vi "Compute ROI Grid v2.vi"(8 "Error In":errorcluster, 10 "Current ROI Bounds":T1, 11 "Grid Definition":T2) -> (0 "Error Out":errorcluster, 1 "ROI Names":string[](array[string]), 3 "Current ROI Descriptor":T4[](array[typedef]) {"Contours"."Type" items=["No Selection", "Point", "Line", "Rectangle", "Oval", "Polygon", "Freehand Region", "Annulus", "Unused2", "Unused3", "Broken Line", "Freehand Line", "Rotated Rectangle"]})   [LabVIEW 2021, in "Image.lvlib"]
uses:
  Image.lvlib
  ROI Grid Definition.ctl
  ROI  Type.ctl
  ROI Bounds.ctl
  <vilib>/Utility/error.llb/Error Cluster From Error Code.vi
  AlliGator/Globals, Variables, Constants/AlliGator Abort.vi
  <vilib>/ErrorRing/Error Ring.xnode
  AlliGator/Globals, Variables, Constants/AlliGator Globals, Variables & Constants.lvlib
  Utilities/Utilities.lvlib
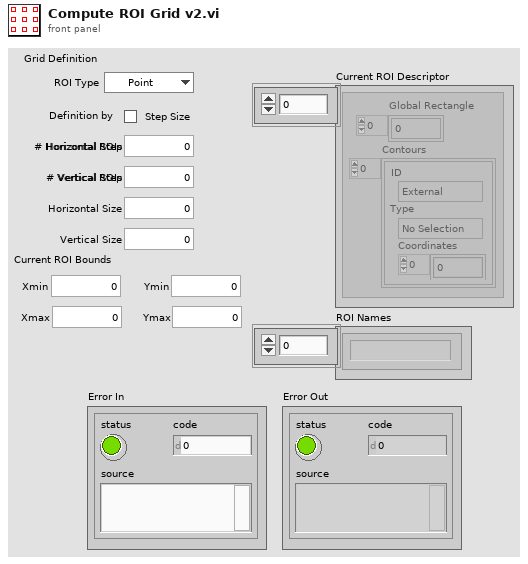
[diagram p1: front panel]
types:
  T1 = typedef "Image.lvlib/ROI Bounds.ctl" = cluster{"Ymax":i32, "Xmin":i32, "Ymin":i32, "Xmax":i32}
  T2 = typedef "Image.lvlib/ROI Grid Definition.ctl" = cluster{"Horizontal Step":i32, "Vertical Step":i32, "Horizontal Size":i32, "Vertical Size":i32, "# Horizontal ROIs":i32, "# Vertical ROIs":i32, "Definition by":bool, "ROI Type":T3}
  T3 = typedef "Image.lvlib/ROI  Type.ctl" = enum16{"Point", "Oval", "Rectangle"}
  T4 = typedef "ROI Descriptor" = cluster{"Global Rectangle":i32[], "Contours":cluster{"ID":enum32{"External", "Internal"}, "Type":u32, "Coordinates":i32[]}[]}
  T5 = typedef "IMAQ Rectangle" = cluster{"Left":i32, "Top":i32, "Right":i32, "Bottom":i32, "Rotation":dbl}
  T6 = typedef "IMAQ Point" = cluster{"X":sgl, "Y":sgl}
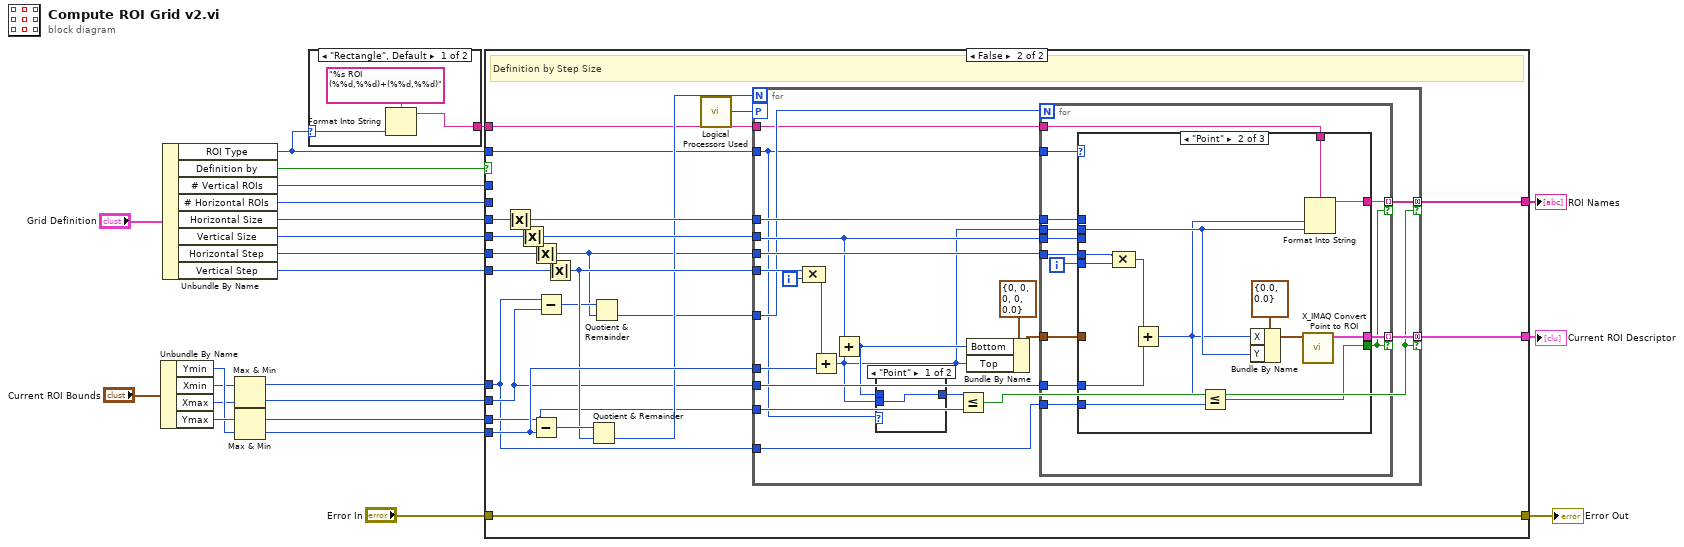
[diagram p0: block diagram]
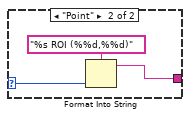
[diagram p2: hidden frame]
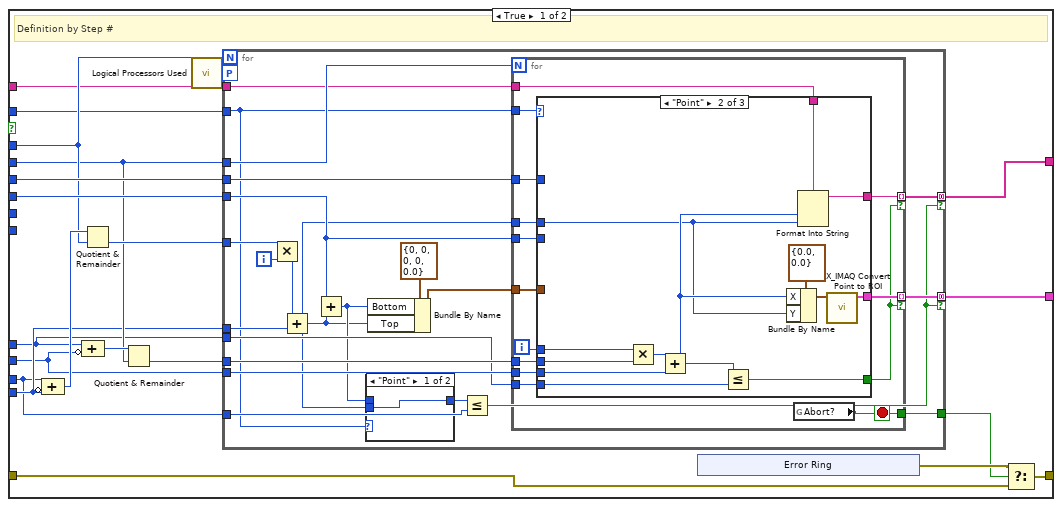
[diagram p3: hidden frame]
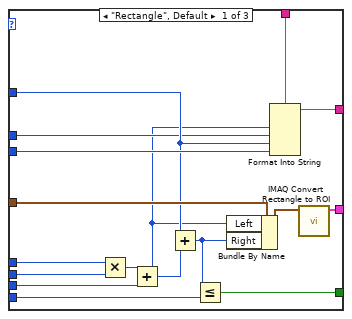
[diagram p5: hidden frame]
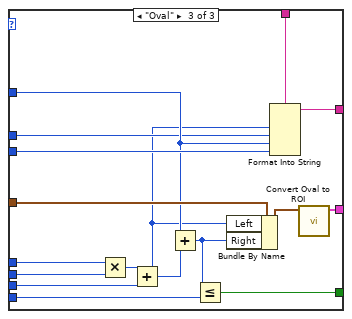
[diagram p6: hidden frame]
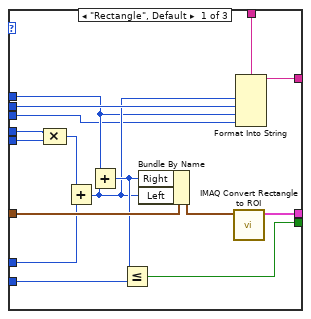
[diagram p8: hidden frame]
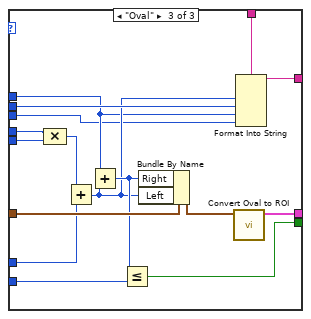
[diagram p9: hidden frame]
diagram:
  n1 = Unbundle By Name("Current ROI Bounds") -> ("Ymin"=w10:i32, "Xmin"=w8:i32, "Xmax"=w7:i32, "Ymax"=w12:i32)
  n2 = Unbundle By Name("Grid Definition") -> ("ROI Type"=w1:T3, "Definition by"=w22:bool, "# Vertical ROIs"=w21:i32, "# Horizontal ROIs"=w18:i32, "Horizontal Size"=w15:i32, "Vertical Size"=w14:i32, "Horizontal Step"=w19:i32, "Vertical Step"=w17:i32)
  n3 = Max & Min(x=w8, y=w7) -> (max(x,y)=w5:i32, min(x,y)=w6:i32)
  n4 = Max & Min(x=w12, y=w10) -> (max(x,y)=w11:i32, min(x,y)=w9:i32)
  n5 = case shown="\"Rectangle\", Default" w1 {
    selector: w1 -> [w24 w27]
    tunnel: [w25 w28] -> w2
    frame "Rectangle", Default {
      n6 = Format Into String(format string="%s ROI (%%d,%%d)+(%%d,%%d)", w24) -> (resulting string=w25:string)  [unwired: 2 in, 1 out]
    }
    frame "Point" {
      n7 = Format Into String(format string="%s ROI (%%d,%%d)", w27) -> (resulting string=w28:string)  [unwired: 2 in, 1 out]
    }
  }
  n8 = case shown="False" w22 {
    tunnel: w21 -> [w45 _]
    tunnel: w19 -> [_ w159]
    tunnel: w6 -> [w35 w146]
    tunnel: w18 -> [w42 _]
    tunnel: w17 -> [_ w158]
    tunnel: w9 -> [w36 w151]
    tunnel: [w50 w157] -> w16
    tunnel: w15 -> [w47 w156]
    tunnel: w14 -> [w49 w155]
    tunnel: w5 -> [w33 w142]
    tunnel: w11 -> [w34 w147]
    tunnel: [w41 w154] -> w13
    tunnel: "Error In" -> [w38 w141]
    tunnel: [w40 w141] -> w3
    tunnel: w2 -> [w32 w140]
    tunnel: w1 -> [w31 w139]
    frame True {
      # "Definition by Step #"
      n9 = Compound Arithmetic op=ADD(w34, invert w36) -> (w46:i32)
      n10 = Compound Arithmetic op=ADD(w33, invert w35) -> (w48:i32)
      n11 = Quotient & Remainder(x=w46, y=w45) -> (floor(x/y)=w44:i32)  [unwired: 1 out]
      n12 = Quotient & Remainder(x=w48, y=w42) -> (floor(x/y)=w43:i32)  [unwired: 1 out]
      n13 = call "Logical Processors Used.vi"() -> ("# Logical Processor Used"=w30:i32)  [unwired: 6 in]
      n14 = for {
        N: w45 -> [_]
        tunnel: w35 -> [w75]
        tunnel: w42 -> [w76]
        tunnel: [w74] -> w50 mode=concatenating if=w61
        tunnel: w47 -> [w73]
        tunnel: w49 -> [w67]
        tunnel: w44 -> [w65]
        tunnel: w43 -> [w70]
        tunnel: [w69] -> w41 mode=concatenating if=w61
        tunnel: [w66] -> w37
        workers-P: w30 -> [_]
        tunnel: w36 -> [w68]
        tunnel: w34 -> [w62]
        tunnel: w33 -> [w60]
        tunnel: w32 -> [w59]
        tunnel: w31 -> [w55]
        i -> [w64]
        n15 = Multiply(x=w65, y=w64) -> (x*y=w63:i32)
        n16 = Add(x=w63, y=w68) -> (x+y=w56:i32)
        n17 = Add(x=w67, y=w56) -> (x+y=w58:i32)
        n18 = case shown="\"Point\"" w55 {
          tunnel: w58 -> [_ w78]
          tunnel: [w77 w78] -> w57
          tunnel: w56 -> [w77 _]
          frame "Point" {
          }
          frame "Oval", Default {
          }
        }
        n19 = Bundle By Name(cluster=T5 {"Left"=0, "Top"=0, "Right"=0, "Bottom"=0, "Rotation"=0.0} ("Rectangle"), "Bottom"=w58, "Top"=w56) -> (w71:T5)
        n20 = Less Or Equal?(x=w57, y=w62) -> (x <= y?=w61:bool)
        n21 = for {
          N: w76 -> [_]
          tunnel: [w92] -> w74 mode=indexing if=w82
          tunnel: w73 -> [w87]
          tunnel: w71 -> [w91]
          tunnel: w70 -> [w85]
          tunnel: [w90] -> w69 mode=indexing if=w82
          tunnel: w67 -> [w88]
          tunnel: [w81] -> w66
          tunnel: w56 -> [w86]
          tunnel: w75 -> [w89]
          tunnel: w60 -> [w83]
          tunnel: w59 -> [w80]
          tunnel: w55 -> [w79]
          i -> [w84]
          stop <- w81 stop-if-true
          n22 = case shown="\"Point\"" w79 {
            tunnel: [w108 w121 w137] -> w92
            tunnel: w91 -> [w107 _ w136]
            tunnel: [w105 w120 w134] -> w90
            tunnel: w89 -> [w104 w119 w133]
            tunnel: w88 -> [w103 _ w132]
            tunnel: w87 -> [w102 _ w131]
            tunnel: w86 -> [w101 w109 w130]
            tunnel: w85 -> [w100 w118 w129]
            tunnel: w84 -> [w99 w117 w128]
            tunnel: w83 -> [w95 w115 w124]
            tunnel: [w94 w114 w123] -> w82
            tunnel: w80 -> [w93 w113 w122]
            frame "Rectangle", Default {
              n23 = Multiply(x=w99, y=w100) -> (x*y=w98:i32)
              n24 = Add(x=w98, y=w104) -> (x+y=w97:i32)
              n25 = Add(x=w102, y=w97) -> (x+y=w96:i32)
              n26 = Less Or Equal?(x=w96, y=w95) -> (x <= y?=w94:bool)
              n27 = Bundle By Name(cluster=w107, "Left"=w97, "Right"=w96) -> (w106:T5)
              n28 = Format Into String(format string=w93, w97, w101, w102, w103) -> (resulting string=w105:string)  [unwired: 2 in, 1 out]
              n29 = call "IMAQ Convert Rectangle to ROI"("Rectangle"=w106) -> ("ROI Descriptor"=w108:T4)  [unwired: 8 in, 1 out]
            }
            frame "Point" {
              n30 = Multiply(x=w117, y=w118) -> (x*y=w116:i32)
              n31 = Add(x=w116, y=w119) -> (x+y=w110:i32)
              n32 = Less Or Equal?(x=w110, y=w115) -> (x <= y?=w114:bool)
              n33 = Bundle By Name(cluster=T6 {"X"=0.0, "Y"=0.0} ("Point"), "X"=w110, "Y"=w109) -> (w111:T6)
              n34 = Format Into String(format string=w113, w110, w109) -> (resulting string=w120:string)  [unwired: 2 in, 1 out]
              n35 = call "X_IMAQ Convert Point to ROI.vi"("Point"=w111) -> ("ROI Descriptor"=w121:T4)  [unwired: 8 in, 1 out]
            }
            frame "Oval" {
              n36 = Multiply(x=w128, y=w129) -> (x*y=w127:i32)
              n37 = Add(x=w127, y=w133) -> (x+y=w126:i32)
              n38 = Add(x=w131, y=w126) -> (x+y=w125:i32)
              n39 = Less Or Equal?(x=w125, y=w124) -> (x <= y?=w123:bool)
              n40 = Bundle By Name(cluster=w136, "Left"=w126, "Right"=w125) -> (w135:T5)
              n41 = Format Into String(format string=w122, w126, w130, w131, w132) -> (resulting string=w134:string)  [unwired: 2 in, 1 out]
              n42 = call "Convert Oval to ROI.vi"("Oval Bounds"=w135) -> ("ROI Descriptor"=w137:T4)  [unwired: 8 in, 1 out]
            }
          }
          n43 = global read "AlliGator Abort.vi" "Abort?"() -> (w81:bool)
        }
      }
      n44 = xnode "Error Ring"() -> ("error out"=w39:errorcluster)
      n45 = Select(t=w39, s=w37, f=w38) -> (s? t:f=w40:errorcluster)
    }
    frame False {
      # "Definition by Step Size"
      n46 = Absolute Value(x=w156) -> (abs(x)=w153:i32)
      n47 = Absolute Value(x=w155) -> (abs(x)=w152:i32)
      n48 = Absolute Value(x=w159) -> (abs(x)=w144:i32)
      n49 = Subtract(x=w147, y=w151) -> (x-y=w150:i32)
      n50 = Subtract(x=w142, y=w146) -> (x-y=w145:i32)
      n51 = Absolute Value(x=w158) -> (abs(x)=w149:i32)
      n52 = Quotient & Remainder(x=w150, y=w149) -> (floor(x/y)=w148:i32)  [unwired: 1 out]
      n53 = Quotient & Remainder(x=w145, y=w144) -> (floor(x/y)=w143:i32)  [unwired: 1 out]
      n54 = call "Logical Processors Used.vi"() -> ("# Logical Processor Used"=w138:i32)  [unwired: 6 in]
      n55 = for {
        N: w148 -> [_]
        tunnel: w144 -> [w178]
        tunnel: w146 -> [w180]
        tunnel: w149 -> [w173]
        tunnel: [w179] -> w157 mode=concatenating if=w165
        tunnel: w153 -> [w177]
        tunnel: w152 -> [w171]
        tunnel: [w172] -> w154 mode=concatenating if=w165
        tunnel: w151 -> [w174]
        tunnel: w147 -> [w168]
        tunnel: w143 -> [w167]
        workers-P: w138 -> [_]
        tunnel: w142 -> [w166]
        tunnel: w140 -> [w164]
        tunnel: w139 -> [w163]
        i -> [w169]
        n56 = Compound Arithmetic op=MULTIPLY(w173, w169) -> (w170:i32)
        n57 = Add(x=w170, y=w174) -> (x+y=w160:i32)
        n58 = Add(x=w171, y=w160) -> (x+y=w162:i32)
        n59 = case shown="\"Point\"" w163 {
          tunnel: w162 -> [_ w182]
          tunnel: [w181 w182] -> w161
          tunnel: w160 -> [w181 _]
          frame "Point" {
          }
          frame "Oval", Default {
          }
        }
        n60 = Less Or Equal?(x=w161, y=w168) -> (x <= y?=w165:bool)
        n61 = Bundle By Name(cluster=T5 {"Left"=0, "Top"=0, "Right"=0, "Bottom"=0, "Rotation"=0.0} ("Rectangle"), "Bottom"=w162, "Top"=w160) -> (w175:T5)
        n62 = for {
          N: w167 -> [_]
          tunnel: [w195] -> w179 mode=indexing if=w188
          tunnel: w178 -> [w190]
          tunnel: w177 -> [w186]
          tunnel: w175 -> [w194]
          tunnel: [w193] -> w172 mode=indexing if=w188
          tunnel: w171 -> [w185]
          tunnel: w180 -> [w191]
          tunnel: w166 -> [w189]
          tunnel: w160 -> [w187]
          tunnel: w164 -> [w184]
          tunnel: w163 -> [w183]
          i -> [w192]
          n63 = case shown="\"Point\"" w183 {
            tunnel: [w211 w224 w240] -> w195
            tunnel: w194 -> [w210 _ w239]
            tunnel: [w208 w223 w237] -> w193
            tunnel: w192 -> [w207 w222 w236]
            tunnel: w191 -> [w205 w220 w234]
            tunnel: w190 -> [w204 w219 w233]
            tunnel: w189 -> [w202 w218 w231]
            tunnel: [w201 w217 w230] -> w188
            tunnel: w187 -> [w200 w213 w229]
            tunnel: w186 -> [w198 _ w227]
            tunnel: w185 -> [w197 _ w226]
            tunnel: w184 -> [w196 w216 w225]
            frame "Rectangle", Default {
              n64 = Compound Arithmetic op=MULTIPLY(w204, w207) -> (w206:i32)
              n65 = Add(x=w206, y=w205) -> (x+y=w199:i32)
              n66 = Add(x=w198, y=w199) -> (x+y=w203:i32)
              n67 = Less Or Equal?(x=w203, y=w202) -> (x <= y?=w201:bool)
              n68 = Bundle By Name(cluster=w210, "Right"=w203, "Left"=w199) -> (w209:T5)
              n69 = call "IMAQ Convert Rectangle to ROI"("Rectangle"=w209) -> ("ROI Descriptor"=w211:T4)  [unwired: 8 in, 1 out]
              n70 = Format Into String(format string=w196, w199, w200, w198, w197) -> (resulting string=w208:string)  [unwired: 2 in, 1 out]
            }
            frame "Point" {
              n71 = Compound Arithmetic op=MULTIPLY(w219, w222) -> (w221:i32)
              n72 = Add(x=w221, y=w220) -> (x+y=w212:i32)
              n73 = Less Or Equal?(x=w212, y=w218) -> (x <= y?=w217:bool)
              n74 = Bundle By Name(cluster=T6 {"X"=0.0, "Y"=0.0} ("Point"), "X"=w212, "Y"=w213) -> (w214:T6)
              n75 = call "X_IMAQ Convert Point to ROI.vi"("Point"=w214) -> ("ROI Descriptor"=w224:T4)  [unwired: 8 in, 1 out]
              n76 = Format Into String(format string=w216, w212, w213) -> (resulting string=w223:string)  [unwired: 2 in, 1 out]
            }
            frame "Oval" {
              n77 = Compound Arithmetic op=MULTIPLY(w233, w236) -> (w235:i32)
              n78 = Add(x=w235, y=w234) -> (x+y=w228:i32)
              n79 = Add(x=w227, y=w228) -> (x+y=w232:i32)
              n80 = Less Or Equal?(x=w232, y=w231) -> (x <= y?=w230:bool)
              n81 = Bundle By Name(cluster=w239, "Right"=w232, "Left"=w228) -> (w238:T5)
              n82 = call "Convert Oval to ROI.vi"("Oval Bounds"=w238) -> ("ROI Descriptor"=w240:T4)  [unwired: 8 in, 1 out]
              n83 = Format Into String(format string=w225, w228, w229, w227, w226) -> (resulting string=w237:string)  [unwired: 2 in, 1 out]
            }
          }
        }
      }
    }
  }
  "Current ROI Descriptor" <- w16
  "Error Out" <- w3
  "ROI Names" <- w13
